vi "ICM aI16.vi"(9 "Swap Bytes":bool, 11 "String In":string) -> (1 "Value I16":i16, 2 "Value":dbl, 3 "String Out":string)   [LabVIEW 2018]
doc: "ICM aI16.vi\n\n This VI is used to parse binary data that contains a I16 integer.\n\nThis VI was original part of the OSDS system.\n\nInstrument Communication Module Version 1.0\nSeptember, 2017 Original Code Consulting David Thomson\n www.originalcode.com"
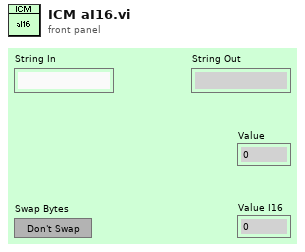
[diagram p1: front panel]
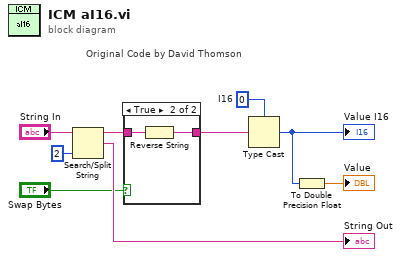
[diagram p0: block diagram]
diagram:
  w7 = i16 0  # I16
  n1 = Search/Split String(string="String In", offset (0)=2) -> (substring before match=w2:string, match + rest of string=→"String Out":string)  [unwired: 2 out]
  n2 = case "Original Code by David Thomson" shown="True" "Swap Bytes" {
    tunnel: w2 -> [w10 w12]
    tunnel: [w10 w11] -> w1
    frame False {
    }
    frame True {
      n3 = Reverse String(1:w12) -> (0:w11:string)
    }
  }
  n4 = Type Cast(type=w7, x=w1) -> (*(type *) &x=w5:i16)
  "Value I16" <- w5
  n5 = To Double Precision Float(number=w5) -> (double precision float=→"Value":dbl)
